vi "VCI_GetRepeaterReference.vi"(8 "error in (no error)":errorcluster caption="错误输入（无错误）", 9 "CANIndex":u32, 10 "DevIndex":u32, 11 "DevType":u32(ring)=2 items=["USB-CAN"=2, "USB-CAN2"=3]) -> (0 "error out":errorcluster caption="错误输出", 2 "On":bool, 3 "Return Val":i32(ring)=1 items=["OK"=1, "ERROR1"=0, "ERROR2"=-1])   [LabVIEW 2011]
uses:
  data/ControlCAN.dll
panel:
  in  "pData":u8[](array[numeric])
  in  "RefType":u8
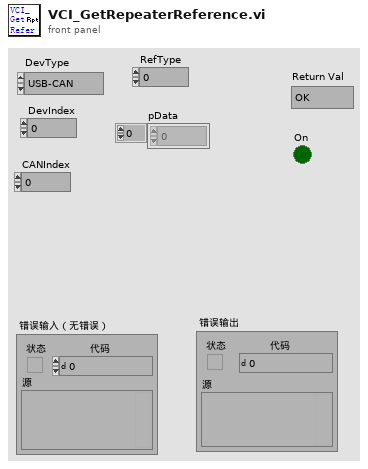
[diagram p1: front panel]
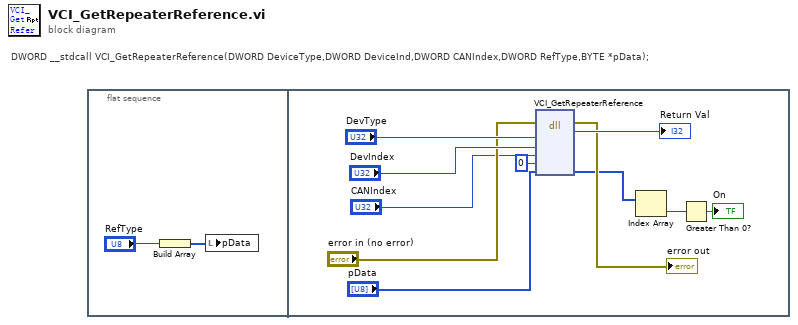
[diagram p0: block diagram]
diagram:
  # "DWORD __stdcall VCI_GetRepeaterReference(DWORD DeviceType,DWORD DeviceInd,DWORD CANIndex,DWORD RefType,BYTE *pData);"
  n1 = flat-sequence {
    frame #0 {
      n2 = Build Array("RefType") -> (w2:u8[])
      n3 = local write "pData"(w2) -> ()
    }
    frame #1 {
      n4 = dll-call lib="PTH1Mabs ZHost_E工作TnewcodeUSB CAN Tool1.98dataControlCAN.dll" fn="VCI_GetRepeaterReference"(error in="error in (no error)", "DevType"="DevType", "DevIndex"="DevIndex", "CANIndex"="CANIndex", "RefType"=u32 0 ("Reserved"), "pData"="pData") -> (error out=→"error out":errorcluster, "ReturnVal"=→"Return Val":i32, "pData"=w7:u8[])  [unwired: 6 in, 1 out]
      n5 = Index Array(array=w7) -> (element=w6:u8)  [unwired: 1 in]
      n6 = Greater Than 0?(x=w6) -> (x > 0?=→"On":bool)
    }
  }
